vi "deleteme.vi"(8 "error in (no error)":errorcluster, 11 "WaveformProcessor in":refnum<class "WaveformProcessor.lvclass">) -> (0 "error out":errorcluster, 3 "WaveformProcessor out":refnum<class "WaveformProcessor.lvclass">)   [LabVIEW 2019, in "Variant Parser.lvlib" / "WaveformProcessor.lvclass"]
uses:
  Library/WaveformProcessor.lvclass
  Library/WaveformProcessor.lvclass/WaveformProcessor.ctl
panel:
  in  "output waveform":waveform(dbl)={"t0"=timestamp(3764754757.690731 s since 1904-01-01), "dt"=2e-06, "Y"=array[10000 elements]}
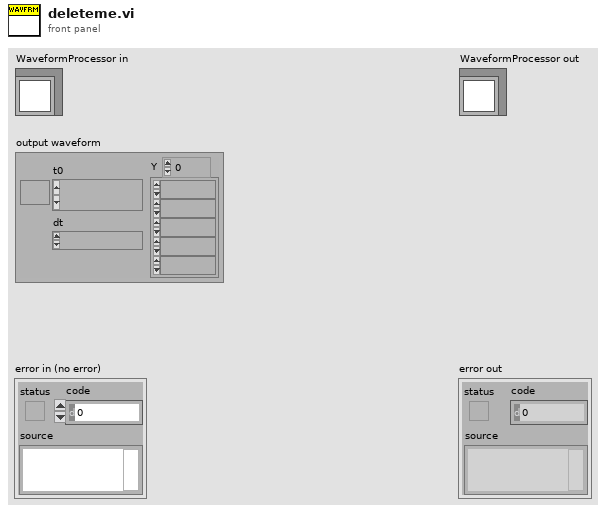
[diagram p1: front panel]
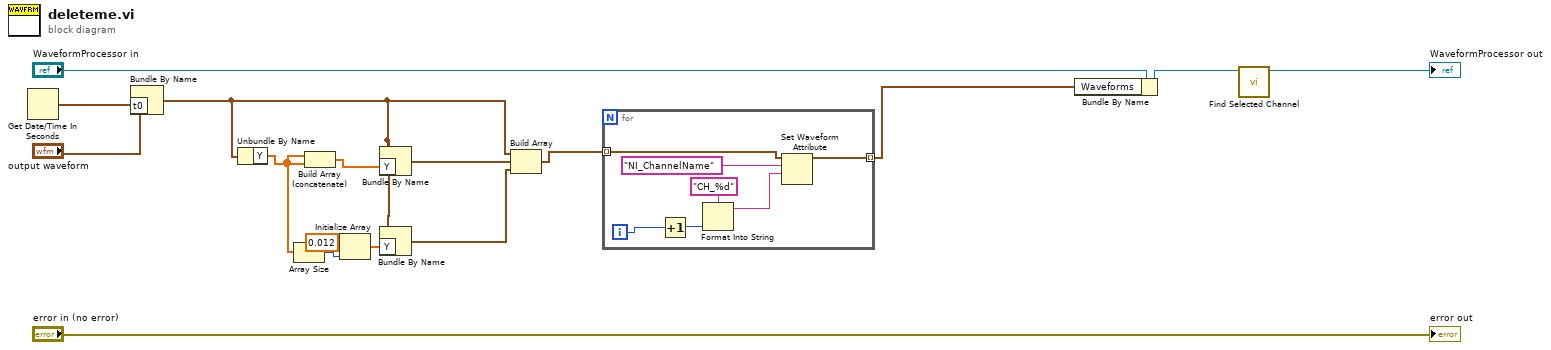
[diagram p0: block diagram]
diagram:
  n1 = Get Date/Time In Seconds() -> (seconds since 1Jan1904=w11:timestamp)
  n2 = Bundle By Name(cluster="output waveform", "t0"=w11) -> (w6:waveform(dbl))
  n3 = Unbundle By Name(w6) -> ("Y"=w5:dbl[])
  n4 = Array Size(array=w5) -> (size(s)=w4:i32)
  n5 = Build Array (concatenate)(w5, w5) -> (w12:dbl[])
  n6 = Initialize Array(0.012 ("element"), w4) -> (w2:dbl[])
  n7 = Bundle By Name(cluster=w6, "Y"=w12) -> (w10:waveform(dbl))
  n8 = Bundle By Name(cluster=w6, "Y"=w2) -> (w1:waveform(dbl))
  n9 = Build Array(w6, w10, w1) -> (w8:waveform(dbl)[])
  n10 = for {
    tunnel: [w20] -> w7 mode=indexing
    tunnel: w8 -> [w17] mode=indexing
    i -> [w23]
    n11 = Increment(x=w23) -> (x+1=w22:i32)
    n12 = Format Into String(format string="CH_%d", w22) -> (resulting string=w19:string)  [unwired: 2 in, 1 out]
    n13 = Set Waveform Attribute(5:w19, 6:"NI_ChannelName" ("name"), 7:w17) -> (3:w20:waveform(dbl))  [unwired: 1 in, 2 out]
  }
  n14 = Bundle By Name(cluster="WaveformProcessor in", "Waveforms"=w7) -> (w9:refnum<class "WaveformProcessor.lvclass">)
  n15 = call "Find Selected Channel.vi"("WaveformProcessor in"=w9) -> ("WaveformProcessor out"=→"WaveformProcessor out":refnum<class "WaveformProcessor.lvclass">)  [unwired: 9 in, 1 out]
  "error out" <- "error in (no error)"
